vi "BenchmarkSystemDefinition.vi"(4 "Tolerance (%)":dbl=3.0 format="%#_13g", 5 "Duration (s)":dbl=30.0 format="%#_13g", 6 "Gateway IP Address (\"\": localhost)":string, 7 "Target Rate List in":dbl[](array[numeric]), 8 "error in (no error)":errorcluster, 9 "overrides files":path[](array[path]), 10 "System Definition File":path, 11 "VeriStandTestCase in":refnum<class "VeriStandTestCase.lvclass">) -> (0 "error out":errorcluster, 3 "VeriStandTestCase out":refnum<class "VeriStandTestCase.lvclass">)   [LabVIEW 2015, in "VeriStandTestCase.lvclass"]
uses:
  VeriStandTestCase.lvclass
  Utilities/BenchmarkInformation.ctl
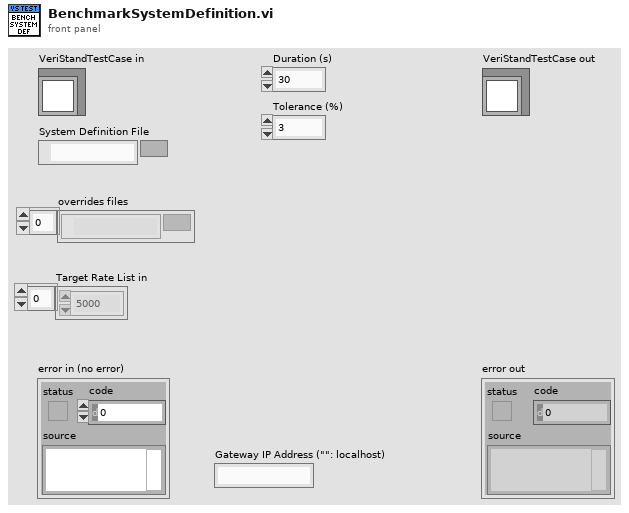
[diagram p1: front panel]
types:
  T1 = typedef "VeriStandTestCase.lvclass/BenchmarkInformation.ctl" = cluster{"Target Rate (Hz)":dbl, "Duration (s)":dbl, "Tolerance (%)":dbl, "Mean Loop Rate (Hz)":dbl, "HP Count":dbl, "Pass?":bool}
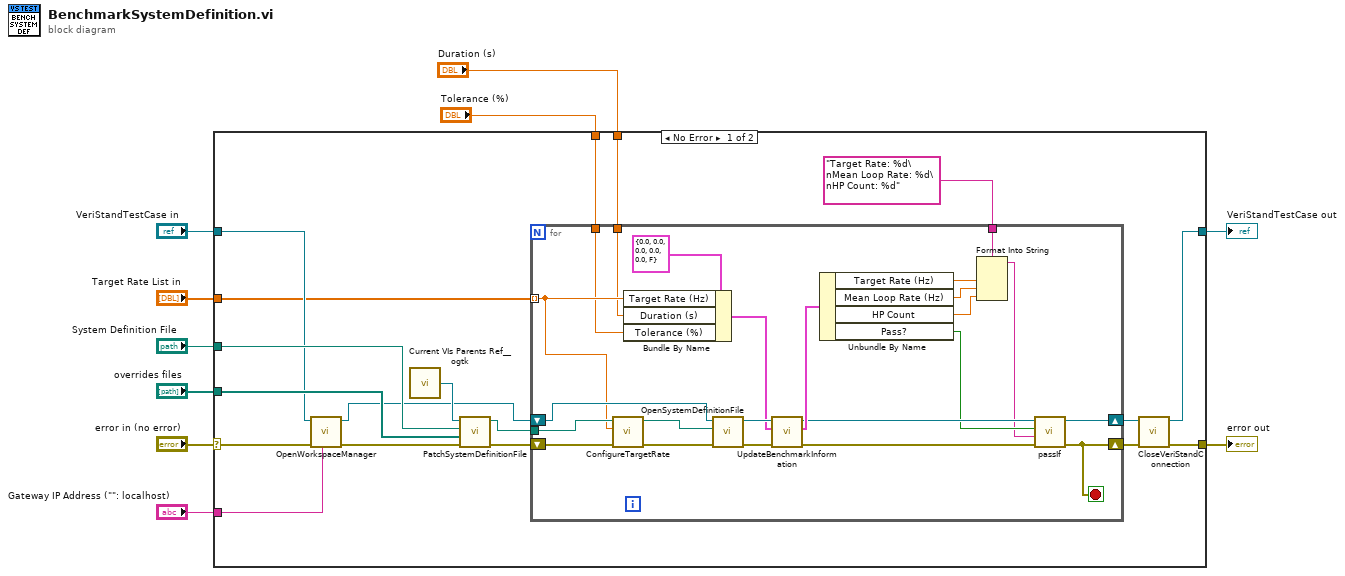
[diagram p0: block diagram]
diagram:
  n1 = case shown="No Error" "error in (no error)" {
    selector: "error in (no error)" -> [w21 w53]
    tunnel: [w23 w53] -> w9
    tunnel: [w17 w52] -> w7
    tunnel: "VeriStandTestCase in" -> [w22 w52]
    tunnel: "Gateway IP Address (\"\": localhost)" -> [w19 _]
    tunnel: "overrides files" -> [w26 _]
    tunnel: "System Definition File" -> [w25 _]
    tunnel: "Target Rate List in" -> [w14 _]
    tunnel: "Duration (s)" -> [w12 _]
    tunnel: "Tolerance (%)" -> [w11 _]
    frame No Error {
      n2 = call "OpenWorkspaceManager.vi"("Gateway IP Address (\"\": localhost)"=w19, "error in (no error)"=w21, "VeriStandTestCase in"=w22) -> ("error out"=w20:errorcluster, "VeriStandTestCase out"=w16:refnum<class "VeriStandTestCase.lvclass">)  [unwired: 7 in]
      n3 = call <userlib>:"Current VIs Parents Ref__ogtk.vi"() -> ("Calling VI's Reference"=w28:refnum<vi>)  [unwired: 2 in]
      n4 = call "PatchSystemDefinitionFile.vi"("error in (no error)"=w20, "overrides files"=w26, "System Definition File"=w25, "VI in"=w28) -> ("error out"=w27:errorcluster, "absolute overridden system definition file"=w24:path)  [unwired: 6 in]
      n5 = for {
        shift-right: [w39] -> w18
        shift-left: w27 -> [w47]
        tunnel: w24 -> [w49]
        shift-right: [w41] -> w15
        shift-left: w16 -> [w50]
        tunnel: w14 -> [w36] mode=indexing
        tunnel: "Target Rate: %d\nMean Loop Rate: %d\nHP Count: %d" ("format string") -> [w35]
        tunnel: w12 -> [w30]
        tunnel: w11 -> [w29]
        stop <- w39 stop-if-true
        n6 = call "ConfigureTargetRate.vi"("error in (no error)"=w47, "Target Rate in"=w36, "absolute overridden system definition file in"=w49) -> ("error out"=w46:errorcluster, "absolute overridden system definition file out"=w48:path)  [unwired: 7 in]
        n7 = Bundle By Name(cluster=T1 {"Target Rate (Hz)"=0.0, "Duration (s)"=0.0, "Tolerance (%)"=0.0, "Mean Loop Rate (Hz)"=0.0, "HP Count"=0.0, "Pass?"=FALSE} ("Benchmark Information"), "Target Rate (Hz)"=w36, "Duration (s)"=w30, "Tolerance (%)"=w29) -> (w37:T1)
        n8 = call "OpenSystemDefinitionFile.vi"("error in (no error)"=w46, "absolute system definition file"=w48, "VeriStand Test Case in"=w50) -> ("error out"=w51:errorcluster, "VeriStand Test Case out"=w44:refnum<class "VeriStandTestCase.lvclass">)  [unwired: 7 in]
        n9 = call "UpdateBenchmarkInformation.vi"("error in (no error)"=w51, "Benchmark Information in"=w37, "VeriStandTestCase in"=w44) -> ("error out"=w45:errorcluster, "Benchmark Information"=w43:T1, "VeriStandTestCase out"=w42:refnum<class "VeriStandTestCase.lvclass">)  [unwired: 6 in]
        n10 = Unbundle By Name(w43) -> ("Target Rate (Hz)"=w34:dbl, "Mean Loop Rate (Hz)"=w33:dbl, "HP Count"=w32:dbl, "Pass?"=w40:bool)
        n11 = Format Into String(format string=w35, w34, w33, w32) -> (resulting string=w31:string)  [unwired: 2 in, 1 out]
        n12 = call-dynamic "passIf.vi"("error in (no error)"=w45, "message (\"\")"=w31, "pass"=w40, "TestCase in"=w42) -> ("error out"=w39:errorcluster, "TestCase out"=w41:refnum<class "VeriStandTestCase.lvclass">)  [unwired: 6 in]
      }
      n13 = call-dynamic "CloseVeriStandConnection.vi"("error in (no error)"=w18, "VeriStand Test Case in"=w15) -> ("error out"=w23:errorcluster, "VeriStand Test Case out"=w17:refnum<class "VeriStandTestCase.lvclass">)  [unwired: 8 in]
    }
    frame Error {
    }
  }
  "error out" <- w9
  "VeriStandTestCase out" <- w7
